vi "MeasureRMS.vi"(2 "# of Samples":dbl, 3 "Sampling Rate":dbl) -> (0 "Waveform Graph":dynamicdata(graph), 1 "RMS":dbl)   [LabVIEW 2015]
panel:
  out "error out":errorcluster
  in  "error in":errorcluster
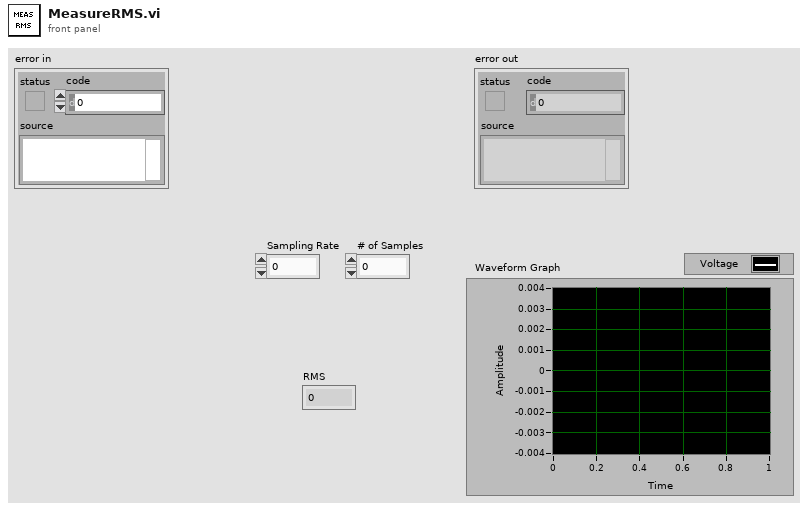
[diagram p1: front panel]
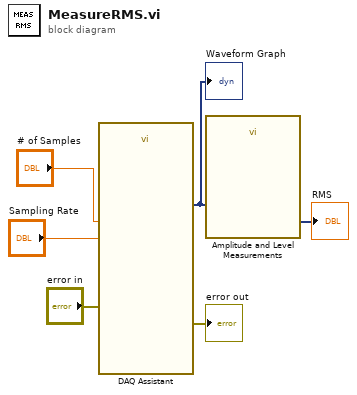
[diagram p0: block diagram]
diagram:
  n1 = call "DAQ Assistant"("rate"="Sampling Rate", "number of samples"="# of Samples", "error in"="error in") -> ("data"=w4:dynamicdata, "error out"=→"error out":errorcluster)  [unwired: 13 in, 2 out]
  "Waveform Graph" <- w4
  n2 = call "Amplitude and Level Measurements"("Signals"=w4) -> ("RMS"=→"RMS":dynamicdata)  [unwired: 13 in, 1 out]
